vi "NIRFSG_ConfigureRF.vi"(6 "Cal Route":string[](array[string])=["", "", ""], 7 "Cal?":bool, 8 "error in (no error)":errorcluster, 9 "Pwr (dBm)":dbl=-90.0 format="%.2f", 10 "Freq (Hz)":dbl=100000000.0 format="%.2p", 11 "RFSG Handle":refnum<k15>) -> (0 "error out":errorcluster, 3 "Adjusted Power Level":dbl)   [LabVIEW 2015]
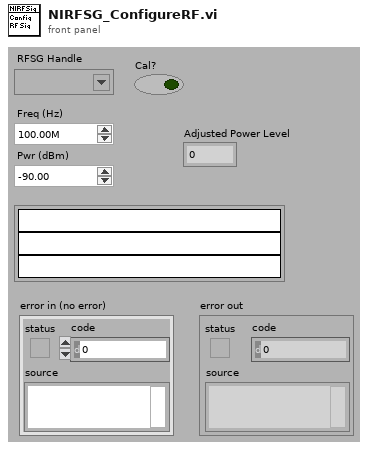
[diagram p1: front panel]
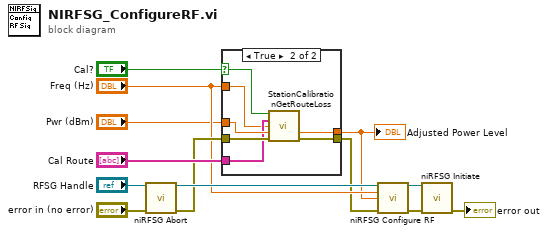
[diagram p0: block diagram]
diagram:
  n1 = call <instrlib>:"niRFSG Abort.vi"("instrument handle"="RFSG Handle", "error in"="error in (no error)") -> ("instrument handle out"=w13:refnum<k15>, "error out"=w6:errorcluster)  [unwired: 12 in]
  n2 = case shown="True" "Cal?" {
    selector: "Cal?" -> [_ w16]
    tunnel: [w14 w22] -> w2
    tunnel: [w15 w17] -> w1
    tunnel: w6 -> [w15 w21]
    tunnel: "Pwr (dBm)" -> [w14 w20]
    tunnel: "Cal Route" -> [_ w19]
    tunnel: "Freq (Hz)" -> [_ w18]
    frame False {
    }
    frame True {
      n3 = call "StationCalibrationGetRouteLoss.vi"("Calibration Enabled"=w16, "Route Names"=w19, "Frequency"=w18, "Power Level"=w20, "error in (no error)"=w21) -> ("Adjusted Power Level"=w22:dbl, "error out"=w17:errorcluster)  [unwired: 7 in, 2 out]
    }
  }
  "Adjusted Power Level" <- w2
  n4 = call <instrlib>:"niRFSG Configure RF.vi"("instrument handle"=w13, "frequency (Hz)"="Freq (Hz)", "power level (dBm)"=w2, "error in"=w1) -> ("instrument handle out"=w12:refnum<k15>, "error out"=w11:errorcluster)  [unwired: 10 in]
  n5 = call <instrlib>:"niRFSG Initiate.vi"("instrument handle"=w12, "error in"=w11) -> ("error out"=→"error out":errorcluster)  [unwired: 12 in, 1 out]
